vi "Read_Double_integer_logic.vi"(10 "Numeric":i32, 11 "register values":u16[](array[numeric])) -> (3 "Array":u16[](array[numeric]))   [LabVIEW 2017]
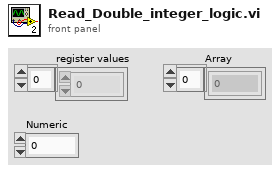
[diagram p1: front panel]
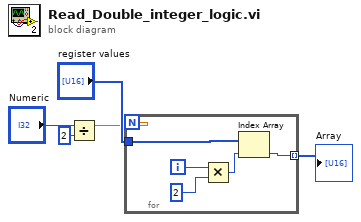
[diagram p0: block diagram]
diagram:
  n1 = Divide(x="Numeric", y=2) -> (x/y=w2:dbl)
  n2 = for {
    N: w2 -> [_]
    tunnel: "register values" -> [w9]
    tunnel: [w6] -> w5 mode=indexing
    i -> [w10]
    n3 = Multiply(x=w10, y=2) -> (x*y=w8:i32)
    n4 = Index Array(array=w9, index=w8) -> (element=w6:u16)
  }
  "Array" <- w5
